vi "Verify MyAnd Parameterized.vi"(11 "Test Case In":refnum<class "Simple Tests.lvclass">) -> (0 "error out":errorcluster, 3 "Test Case Out":refnum<class "Simple Tests.lvclass">)   [LabVIEW 2020, in "Simple Tests.lvclass"]
uses:
  Simple Tests.lvclass
  C:/Program Files/National Instruments/LabVIEW 2026/vi.lib/Astemes/LUnit/Test Case.lvclass
  Simple Tests.lvclass/Simple Tests.ctl
  <vilib>/SAS/Approval Tests/Extensions/LUnit.Extension/lib_LUnit.Extension.lvlib
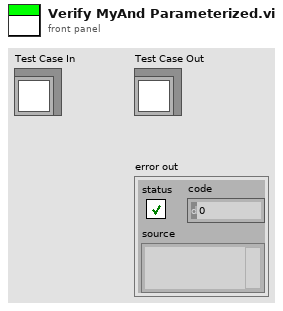
[diagram p1: front panel]
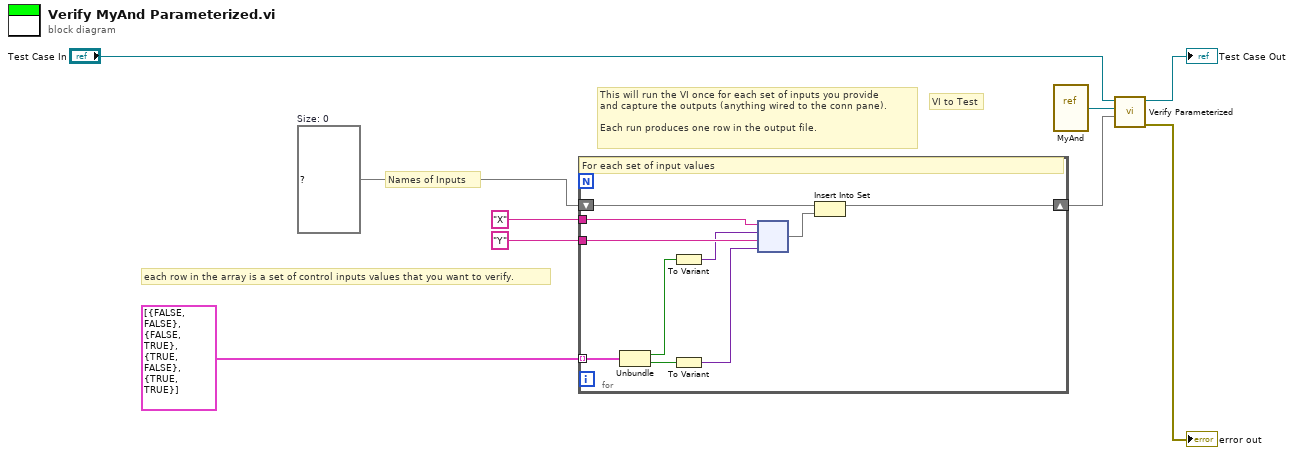
[diagram p0: block diagram]
diagram:
  w7 = set{map{string, variant}} {}  # Size: 0
  # "This will run the VI once for each set of inputs you provide\nand capture the outputs (anything wired to the conn pane).\n\nEach run produces one row in the output file."
  # "VI to Test"
  # "each row in the array is a set of control inputs values that you want to verify."
  # "Names of Inputs"
  n1 = for {
    tunnel: "X" -> [w19]
    tunnel: cluster{bool, bool}[] [{FALSE, FALSE}, {FALSE, TRUE}, {TRUE, FALSE}, {TRUE, TRUE}] -> [w17] mode=indexing
    tunnel: "Y" -> [w18]
    shift-right: [w11] -> w8
    shift-left: w7 -> [w10]
    # "For each set of input values"
    n2 = Unbundle(w17) -> (w16:bool, w15:bool)
    n3 = To Variant(anything=w16) -> (Variant=w13:variant)
    n4 = To Variant(anything=w15) -> (Variant=w12:variant)
    n5 = node(w19, w13, w18, w12) -> (w14:map{string, variant})
    n6 = Insert Into Set(10:w14, 11:w10) -> (3:w11:set{map{string, variant}})  [unwired: 1 out]
  }
  n7 = vi-ref "MyAnd.vi"() -> (w3:refnum<vi>)
  n8 = call <vilib>:"Verify Parameterized.vi"("Set of ctl label -> value var"=w8, "VI in"=w3, "LUnit Test Case In"="Test Case In") -> ("error out"=→"error out":errorcluster, "LUnit Test Case Out"=→"Test Case Out":refnum<class "Simple Tests.lvclass">)  [unwired: 7 in]
